vi "总磷启动流程.vi"() -> ()   [LabVIEW 2016]
uses:
  <vilib>/Utility/miscctls.llb/LVPointTypeDef.ctl
panel:
  out "加标回收实测值":sgl
  out "加标回收数据时间":timestamp
  out "跨度核查实测值":sgl
  out "跨度核查数据时间":timestamp
  out "空白实测值":sgl
  out "空白数据时间":timestamp
  out "水样实测值":sgl
  out "水样数据时间":timestamp
  out "启动记录":string
  out "流程运行中":bool
  out "启动次数":i32
  out "日期/时间":string
  out "运行状态":string
  out "步骤运行时间/秒":i32
  out "流程结束":bool
  out "当前步骤":T1(ring)
  in  "步骤时间/秒":T2={"步骤1时间"=2, "步骤2时间"=4, "步骤3时间"=2, "步骤4时间"=5, "步骤5时间"=6, "步骤6时间"=3, "步骤7时间"=4, "步骤8时间"=7, "步骤9时间"=8, "步骤10时间"=6}
  # "总磷模块"
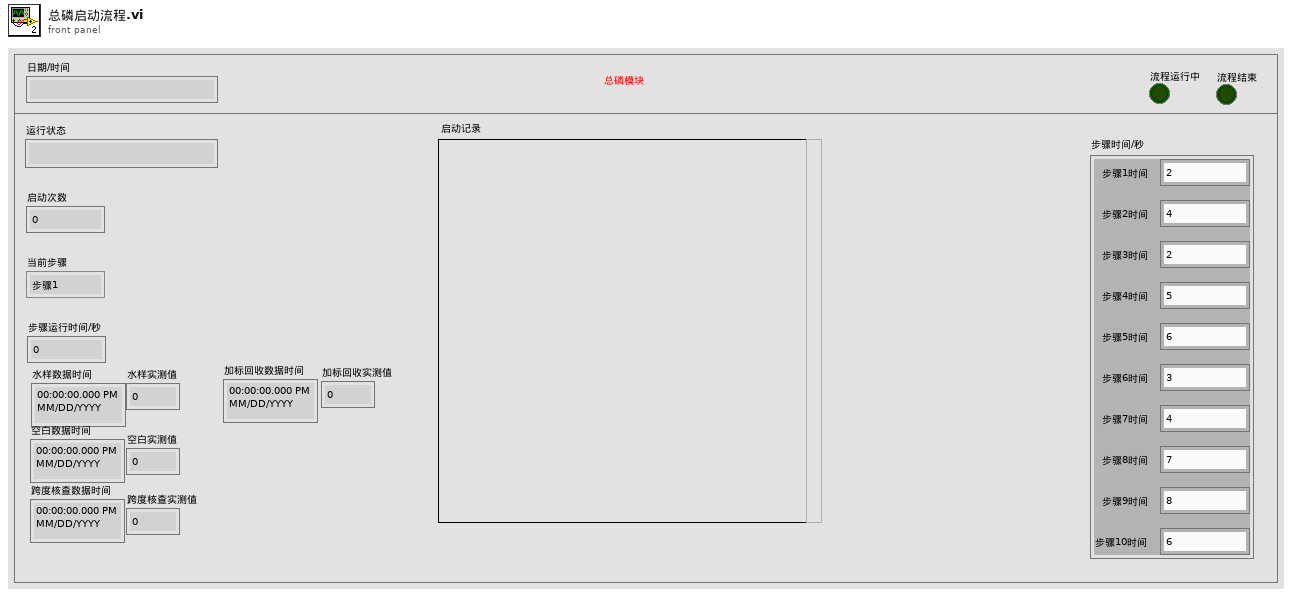
[diagram p1: front panel]
types:
  T1 = enum16{"步骤1", "步骤2", "步骤3", "步骤4", "步骤5", "步骤6", "步骤7", "步骤8", "步骤9", "步骤10"}
  T2 = cluster{"步骤1时间":i32, "步骤2时间":i32, "步骤3时间":i32, "步骤4时间":i32, "步骤5时间":i32, "步骤6时间":i32, "步骤7时间":i32, "步骤8时间":i32, "步骤9时间":i32, "步骤10时间":i32}
  T3 = enum16{"write register", "read register", "write and read register", "write coil", "read coil"}
  T4 = typedef "LVPointTypeDef.ctl" = cluster{"Horizontal":i16, "Vertical":i16}
  T5 = enum32{"Bad", "Idle", "Run top level", "Running"}
  T6 = cluster{"系统时间":timestamp, "工作状态":u16, "测量模式":u16, "告警代码":enum16{"无告警", "缺试剂告警", "缺水样告警", "缺蒸馏水告警", "缺标液告警", "仪表漏液告警", "标定异常告警", "超量程告警", "加热异常", "低试剂预警", "超上限告警", "超下限告警", "仪表内部其他异常", "滴定异常告警", "电极异常告警", "量程切换告警", "参数设置告警", "PH电极电位异常", "电导率电极异常", "浊度光度异常", "溶解氧电极异常", "溶解氧光强异常", "温度异常告警", "PH异常告警", "溶解氧异常告警", "电导率异常告警", "浊度异常告警", "叶绿素异常告警", "藻密度异常告警", "蓝绿藻异常告警", "ORP异常告警", "氨氮异常告警", "清洁刷异常告警", "SD卡异常告警", "蓝牙异常告警", "Wifi异常告警", "流程异常告警"}, "故障代码":enum16{"无故障", "电机故障", "温度故障", "通讯故障", "滴定故障"}, "日志代码":u16, "软件版本":u16, "F0":sgl, "F1":sgl, "F2":sgl, "F3":sgl, "T":sgl, "H":sgl, "id":u16, "flowid":u16, "量程":u16}
  T7 = cluster{"因子编码":u32, "单位":u16, "标样参考值":sgl, "水样数据时间":timestamp, "水样实测值":sgl, "水样数据标识":string, "标样数据时间":timestamp, "标样实测值":sgl, "标样数据标识":string, "空白数据时间":timestamp, "空白实测值":sgl, "空白数据标识":string, "零点核查数据时间":timestamp, "零点核查实测值":sgl, "零点核查数据标识":string, "跨度核查数据时间":timestamp, "跨度核查实测值":sgl, "跨度核查数据标识":string, "加标回收数据时间":timestamp, "加标回收实测值":sgl, "加标回收数据标识":string, "平行样数据时间":timestamp, "平行样实测值":sgl, "平行样数据标识":string}
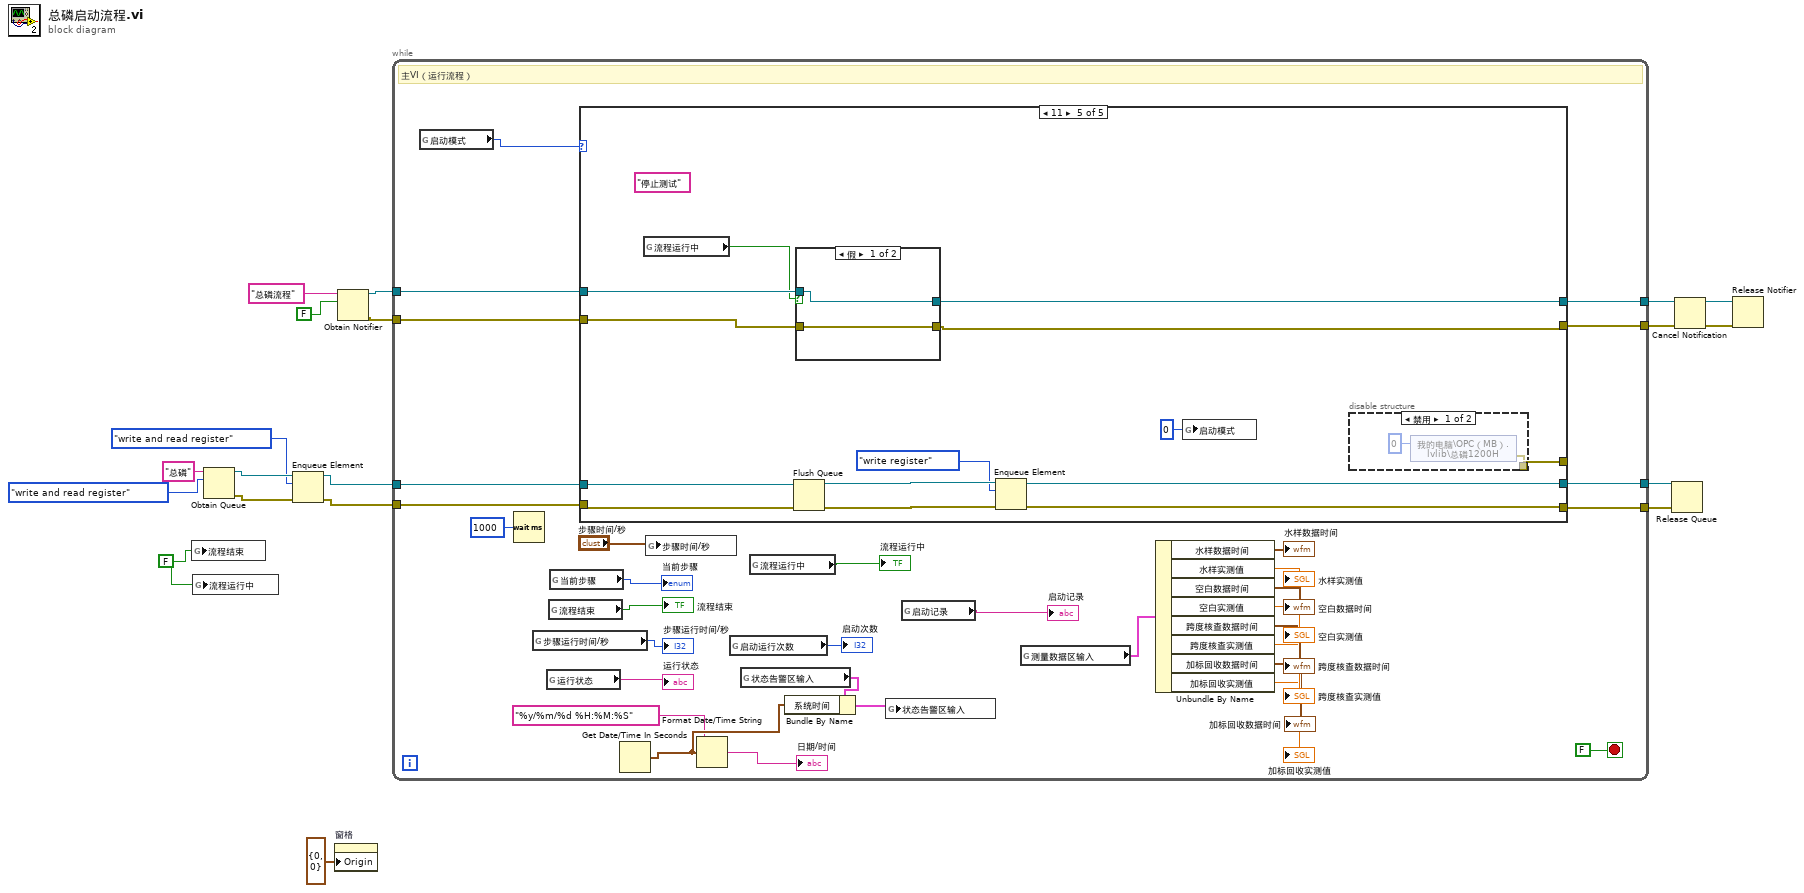
[diagram p0: block diagram]
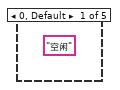
[diagram p2: hidden frame]
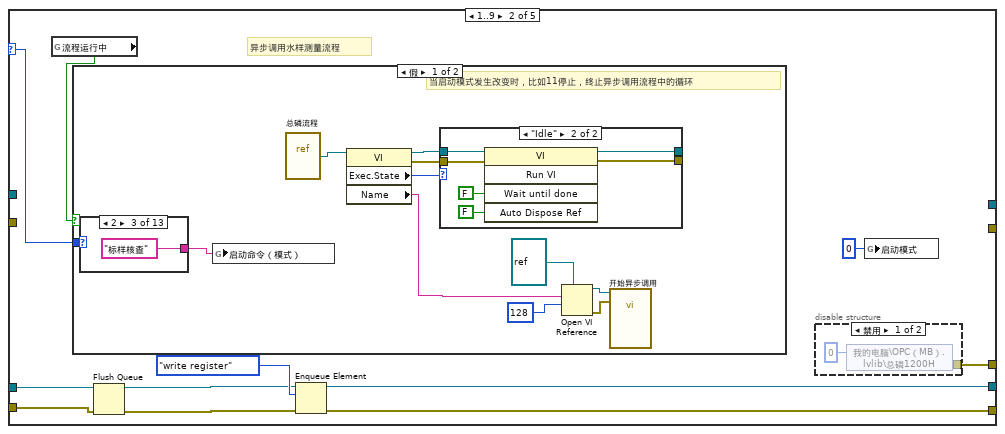
[diagram p3: hidden frame]
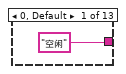
[diagram p5: hidden frame]
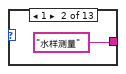
[diagram p6: hidden frame]
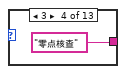
[diagram p7: hidden frame]
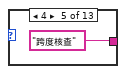
[diagram p8: hidden frame]
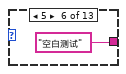
[diagram p9: hidden frame]
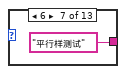
[diagram p10: hidden frame]
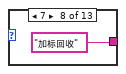
[diagram p11: hidden frame]
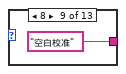
[diagram p12: hidden frame]
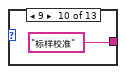
[diagram p13: hidden frame]
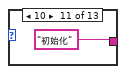
[diagram p14: hidden frame]
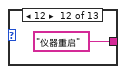
[diagram p15: hidden frame]
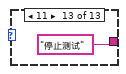
[diagram p16: hidden frame]
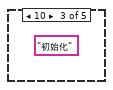
[diagram p19: hidden frame]
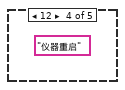
[diagram p20: hidden frame]
diagram:
  w10 = FALSE ("流程结束")
  n1 = global write "总磷全局.vi" "流程结束"(w10) -> ()
  n2 = global write "总磷全局.vi" "流程运行中"(w10) -> ()
  n3 = Obtain Queue(name (unnamed)="总磷" ("名称（未命名）"), element data type=T3."write and read register") -> (queue out=w7:refnum<queue>, error out=w6:errorcluster)  [unwired: 3 in, 1 out]
  n4 = Enqueue Element(queue=w7, element=T3."write and read register", error in (no error)=w6) -> (queue out=w4:refnum<queue>, error out=w3:errorcluster)  [unwired: 1 in, 1 out]
  n5 = property on="窗格" class="Pane"("Origin"=T4 {"Horizontal"=0, "Vertical"=0} ("原点")) -> ()  [unwired: 2 in, 2 out]
  n6 = Obtain Notifier(name (unnamed)="总磷流程" ("名称（未命名）"), notification data type=FALSE) -> (notifier out=w15:refnum<notifier>, error out=w14:errorcluster)  [unwired: 2 in, 1 out]
  n7 = while {
    tunnel: w14 -> [w50]
    tunnel: w15 -> [w49]
    tunnel: [w48] -> w18
    tunnel: [w47] -> w19
    tunnel: w4 -> [w23]
    tunnel: w3 -> [w22]
    tunnel: [w21] -> w2
    tunnel: [w20] -> w1
    stop <- FALSE stop-if-true
    # "主VI（运行流程）"
    n8 = global read "总磷全局.vi" "启动模式"() -> (w24:u16)
    n9 = Wait (ms)(milliseconds to wait=u32 1000 ("等待时间（毫秒）")) -> ()  [unwired: 1 out]
    n10 = global read "总磷全局.vi" "步骤运行时间/秒"() -> (→"步骤运行时间/秒":i32)
    n11 = global read "总磷全局.vi" "运行状态"() -> (→"运行状态":string)
    n12 = global read "总磷全局.vi" "流程结束"() -> (→"流程结束":bool)
    n13 = global read "总磷全局.vi" "当前步骤"() -> (→"当前步骤":T1)
    n14 = case shown="11" w24 {
      selector: w24 -> [_ w63 _ _ _]
      tunnel: w50 -> [_ _ _ _ w111]
      tunnel: w49 -> [_ _ _ _ w110]
      tunnel: [_ _ _ _ w109] -> w48
      tunnel: [_ _ _ _ w108] -> w47
      tunnel: [_ w61 _ _ w106] -> _
      tunnel: w23 -> [_ w56 _ _ w101]
      tunnel: w22 -> [_ w55 _ _ w100]
      tunnel: [_ w54 _ _ w99] -> w21
      tunnel: [_ w53 _ _ w98] -> w20
      frame 0, Default {
        (unwired) "空闲"
      }
      frame 1..9 {
        # "异步调用水样测量流程"
        n15 = global read "总磷全局.vi" "流程运行中"() -> (w62:bool)
        n16 = case shown="假" w62 {
          tunnel: w63 -> [w67 _]
          frame False {
            # "当启动模式发生改变时，比如11停止，终止异步调用流程中的循环"
            n17 = case shown="2" w67 {
              tunnel: ["空闲" "水样测量" "标样核查" "零点核查" "跨度核查" "空白测试" "平行样测试" "加标回收" "空白校准" "标样校准" "初始化" "仪器重启" "停止测试"] -> w66
              frame 0, Default {
              }
              frame 1 {
              }
              frame 2 {
              }
              frame 3 {
              }
              frame 4 {
              }
              frame 5 {
              }
              frame 6 {
              }
              frame 7 {
              }
              frame 8 {
              }
              frame 9 {
              }
              frame 10 {
              }
              frame 12 {
              }
              frame 11 {
              }
            }
            n18 = global write "总磷全局.vi" "启动命令（模式）"(w66) -> ()
            n19 = vi-ref "总磷流程.vi"() -> (w76:refnum<vi>)
            n20 = property class="VI"(reference=w76) -> (reference out=w75:refnum<vi>, error out=w73:errorcluster, "Exec.State"=w74:T5, "Name"=w68:string)  [unwired: 1 in]
            n21 = case shown="\"Idle\"" w74 {
              tunnel: w75 -> [w91 w97]
              tunnel: [w91 w96] -> _
              tunnel: w73 -> [w90 w93]
              tunnel: [w90 w92] -> _
              frame "Bad", Default {
              }
              frame "Idle" {
                n22 = invoke class="VI" method="Run VI"(reference=w97, error in=w93, "Wait until done"=FALSE ("结束前等待"), "Auto Dispose Ref"=FALSE ("自动销毁引用")) -> (reference out=w96:refnum<vi>, error out=w92:errorcluster)  [unwired: 1 in, 3 out]
              }
            }
            n23 = Open VI Reference(type specifier VI Refnum (for type only)=refnum<vi> refnum ("类型说明符VI引用句柄（仅用于类型）"), vi path=w68, options=128 ("选项")) -> (vi reference=w72:refnum<vi>, error out=w70:errorcluster)  [unwired: 3 in]
            n24 = call-by-ref "开始异步调用"(reference=w72, error in=w70) -> ()  [unwired: 12 in, 2 out]
          }
          frame True {
          }
        }
        n25 = Flush Queue(queue=w56, error in (no error)=w55) -> (queue out=w57:refnum<queue>, error out=w58:errorcluster)  [unwired: 1 out]
        n26 = Enqueue Element(queue=w57, element=T3."write register", error in (no error)=w58) -> (queue out=w54:refnum<queue>, error out=w53:errorcluster)  [unwired: 1 in, 1 out]
        n27 = disable-structure shown="禁用" {
          disable-tunnel: [w64 _] -> w61
          frame Disabled {
            n28 = shared-variable "我的电脑\\OPC（MB）.lvlib\\总磷1200H"(u16 0 ("总磷1200H")) -> (error out=w64:errorcluster)  [unwired: 1 in]
          }
          frame Enabled {
          }
        }
        n29 = global write "总磷全局.vi" "启动模式"(u16 0 ("启动模式")) -> ()
      }
      frame 10 {
        (unwired) "初始化"
      }
      frame 12 {
        (unwired) "仪器重启"
      }
      frame 11 {
        (unwired) "停止测试"
        n30 = global read "总磷全局.vi" "流程运行中"() -> (w107:bool)
        n31 = Flush Queue(queue=w101, error in (no error)=w100) -> (queue out=w104:refnum<queue>, error out=w103:errorcluster)  [unwired: 1 out]
        n32 = case shown="假" w107 {
          tunnel: w111 -> [w114 w119]
          tunnel: w110 -> [w115 w118]
          tunnel: [w115 w117] -> w109
          tunnel: [w114 w116] -> w108
          frame False {
          }
          frame True {
            n33 = Send Notification(notification=TRUE ("通知"), notifier=w118, error in (no error)=w119) -> (notifier out=w117:refnum<notifier>, error out=w116:errorcluster)
          }
        }
        n34 = Enqueue Element(queue=w104, element=T3."write register", error in (no error)=w103) -> (queue out=w99:refnum<queue>, error out=w98:errorcluster)  [unwired: 1 in, 1 out]
        n35 = global write "总磷全局.vi" "启动模式"(u16 0 ("启动模式")) -> ()
        n36 = disable-structure shown="禁用" {
          disable-tunnel: [w112 _] -> w106
          frame Disabled {
            n37 = shared-variable "我的电脑\\OPC（MB）.lvlib\\总磷1200H"(u16 0 ("总磷1200H")) -> (error out=w112:errorcluster)  [unwired: 1 in]
          }
          frame Enabled {
          }
        }
      }
    }
    n38 = Get Date/Time In Seconds() -> (seconds since 1Jan1904=w46:timestamp)
    n39 = global write "总磷全局.vi" "步骤时间/秒"("步骤时间/秒") -> ()
    n40 = Format Date/Time String(time format string (%c)="%y/%m/%d %H:%M:%S" ("时间格式字符串(%c)"), seconds (now)=w46) -> (date/time string=→"日期/时间":string)  [unwired: 1 in]
    n41 = global read "总磷全局.vi" "启动运行次数"() -> (→"启动次数":i32)
    n42 = global read "总磷全局.vi" "状态告警区输入"() -> (w42:T6)
    n43 = global read "总磷全局.vi" "流程运行中"() -> (→"流程运行中":bool)
    n44 = Bundle By Name(cluster=w42, "系统时间"=w46) -> (w43:T6)
    n45 = global write "总磷全局.vi" "状态告警区输入"(w43) -> ()
    n46 = global read "总磷全局.vi" "启动记录"() -> (→"启动记录":string)
    n47 = global read "总磷全局.vi" "测量数据区输入"() -> (w33:T7)
    n48 = Unbundle By Name(w33) -> ("水样数据时间"=→"水样数据时间":timestamp, "水样实测值"=→"水样实测值":sgl, "空白数据时间"=→"空白数据时间":timestamp, "空白实测值"=→"空白实测值":sgl, "跨度核查数据时间"=→"跨度核查数据时间":timestamp, "跨度核查实测值"=→"跨度核查实测值":sgl, "加标回收数据时间"=→"加标回收数据时间":timestamp, "加标回收实测值"=→"加标回收实测值":sgl)
  }
  n49 = Release Queue(queue=w2, error in (no error)=w1) -> ()  [unwired: 1 in, 3 out]
  n50 = Cancel Notification(0:w18, 3:w19) -> (8:w17:refnum<notifier>, 11:w16:errorcluster)  [unwired: 1 out]
  n51 = Release Notifier(notifier=w17, error in (no error)=w16) -> ()  [unwired: 1 in, 3 out]
